vi "Enqueue.vi"(5 "QueName":string="BaseVisQue", 7 "Priority? (F)":bool, 8 "Error":errorcluster[](array[cluster]), 9 "Data":variant, 10 "Message":string) -> (0 "Error":errorcluster[](array[cluster]))   [LabVIEW 2014, in "Visualization.lvlib" / "VisualizeBase.lvclass"]
uses:
  VisualizeBase/VisualizeBase_class/VisualizeBase.lvclass
  Typedefs/MsgType.ctl
  <userlib>/NIST/NISTErrorLib/NISTErrorLib.lvlib
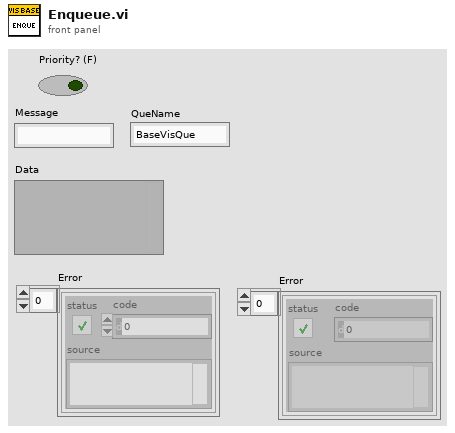
[diagram p1: front panel]
types:
  T1 = typedef "Visualization.lvlib/VisualizeBase.lvclass/MsgType.ctl" = cluster{"Message":string, "Data":variant}
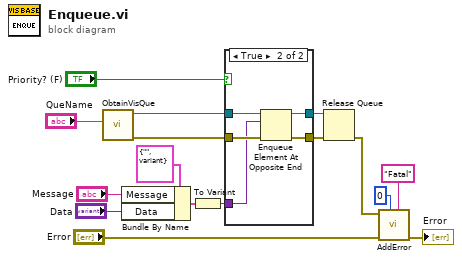
[diagram p0: block diagram]
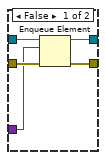
[diagram p2: hidden frame]
diagram:
  n1 = call "ObtainVisQue.vi"("QueName"="QueName") -> ("error out"=w11:errorcluster, "queue out"=w15:refnum<queue>)  [unwired: 9 in]
  n2 = Bundle By Name(cluster=T1 {"Message"="", "Data"=variant} ("clMsgType"), "Message"="Message", "Data"="Data") -> (w10:T1)
  n3 = To Variant(anything=w10) -> (Variant=w9:variant)
  n4 = case shown="True" "Priority? (F)" {
    tunnel: w15 -> [w20 w26]
    tunnel: w11 -> [w21 w25]
    tunnel: w9 -> [w19 w24]
    tunnel: [w18 w23] -> w2
    tunnel: [w17 w22] -> w3
    frame False {
      n5 = Enqueue Element(queue=w20, element=w19, error in (no error)=w21) -> (queue out=w17:refnum<queue>, error out=w18:errorcluster)  [unwired: 1 in, 1 out]
    }
    frame True {
      n6 = Enqueue Element At Opposite End(queue=w26, element=w24, error in (no error)=w25) -> (queue out=w22:refnum<queue>, error out=w23:errorcluster)  [unwired: 1 in, 1 out]
    }
  }
  n7 = Release Queue(queue=w3, error in (no error)=w2) -> (error out=w1:errorcluster)  [unwired: 1 in, 2 out]
  n8 = call <userlib>:"AddError.vi"("Severity"="Fatal" ("String"), "Priority"=u8 0, "ErrorArray"="Error", "error in (no error)"=w1) -> ("ErrorArray"=→"Error":errorcluster[])  [unwired: 6 in, 1 out]
